vi "Stabilizing.vi"(4 "output cluster":T10, 5 "Max Humidity Wait Time":i32, 10 "output cluster 3":T2 {"Current Settings"."Pump" items=["Pump 0", "Pump 1", "Pump 2", "Pump 3", "Pump 4", "Pump 5"]; "Current Settings"."Chart X axis Timescale" min=20 max=180 step=1; "Current Settings"."RunTime Mode Settings"."Exp. Gas Tank" items=["0.07", "0.031", "0.877", "1.863", "3.881", "5.790", "7.688", "6.000"]; "Current Settings"."RunTime Mode Settings"."Insp. Gas Tank" items=["0.07", "0.031", "0.877", "1.863", "3.881", "5.790", "7.688", "6.000"]; "Current Settings"."RunTime Mode Settings"."I:E Ratio" max=30 scale=0.0..7.0; "Current Settings"."RunTime Mode Settings"."Resp Rate Brpm" min=0 max=30 format="%.2f"; "Current Settings"."TE#2 Configuration"."Serial Port"."XOFF Char" format="%.0x"; "Current Settings"."TE#2 Configuration"."Serial Port"."XON Char" format="%.0x"; "Current Settings"."TE#2 Configuration"."Serial Port"."flow control" items=["None"=0, "XON/XOFF"=1, "RTS/CTS"=2, "DTR/DSR"=4]; "Current Settings"."TE#2 Configuration"."Serial Port"."stop bits" items=["1.0"=10, "1.5"=15, "2.0"=20]; "Current Settings"."TE#2 Configuration"."Serial Port"."data bits" min=5 max=8 step=1; "Current Settings"."TE#2 Configuration"."Serial Port"."baud rate" items=["75"=75, "110"=110, "134"=134, "150"=150, "300"=300, "600"=600, "1200"=1200, "1800"=1800, "2400"=2400, "4800"=4800, "7200"=7200, "9600"=9600, "14400"=14400, "19200"=19200, "28800"=28800, "38400"=38400, "56000"=56000, "57600"=57600, "115200"=115200, "128000"=128000, "230400"=230400]; "Current Settings"."TE#2 Configuration"."Serial Port"."termination char" format="%.0x"; "Current Settings"."TE#1 Configuration"."Serial Port"."XOFF Char" format="%.0x"; "Current Settings"."TE#1 Configuration"."Serial Port"."XON Char" format="%.0x"; "Current Settings"."TE#1 Configuration"."Serial Port"."flow control" items=["None"=0, "XON/XOFF"=1, "RTS/CTS"=2, "DTR/DSR"=4]; "Current Settings"."TE#1 Configuration"."Serial Port"."stop bits" items=["1.0"=10, "1.5"=15, "2.0"=20]; "Current Settings"."TE#1 Configuration"."Serial Port"."data bits" min=5 max=8 step=1; "Current Settings"."TE#1 Configuration"."Serial Port"."baud rate" items=["75"=75, "110"=110, "134"=134, "150"=150, "300"=300, "600"=600, "1200"=1200, "1800"=1800, "2400"=2400, "4800"=4800, "7200"=7200, "9600"=9600, "14400"=14400, "19200"=19200, "28800"=28800, "38400"=38400, "56000"=56000, "57600"=57600, "115200"=115200, "128000"=128000, "230400"=230400]; "Current Settings"."TE#1 Configuration"."Serial Port"."termination char" format="%.0x"; "Current Settings"."Capnometer Configuration"."Device" items=["None", "TidalWave", "LoFlow / Canary", "Capnogard"]; "Current Settings"."Capnometer Configuration"."Serial Port"."XOFF Char" format="%.0x"; "Current Settings"."Capnometer Configuration"."Serial Port"."XON Char" format="%.0x"; "Current Settings"."Capnometer Configuration"."Serial Port"."flow control" items=["None"=0, "XON/XOFF"=1, "RTS/CTS"=2, "DTR/DSR"=4]; "Current Settings"."Capnometer Configuration"."Serial Port"."stop bits" items=["1.0"=10, "1.5"=15, "2.0"=20]; "Current Settings"."Capnometer Configuration"."Serial Port"."data bits" min=5 max=8 step=1; "Current Settings"."Capnometer Configuration"."Serial Port"."baud rate" items=["75"=75, "110"=110, "134"=134, "150"=150, "300"=300, "600"=600, "1200"=1200, "1800"=1800, "2400"=2400, "4800"=4800, "7200"=7200, "9600"=9600, "14400"=14400, "19200"=19200, "28800"=28800, "38400"=38400, "56000"=56000, "57600"=57600, "115200"=115200, "128000"=128000, "230400"=230400]; "Current Settings"."Capnometer Configuration"."Serial Port"."termination char" format="%.0x"; "Current Settings"."DAQx Settings"."Analog Output Settings (Volts)" format="%#.3g"; "Current Settings"."DAQx Settings"."Duty Cycle" min=10.0 max=90.0 format="%.1g"; "Current Settings"."DAQx Settings"."Frequency" min=20.0 max=200.0; "Current Settings"."DataLogging Settings"."Data File Duration (Minutes)" min=2 max=200 format="%#.2g"; "Current Settings"."Calibration Settings"."Tolerance #2" min=2 max=4096; "Current Settings"."Calibration Settings"."Cal. Average" min=2 max=4096; "Current Settings"."Test Settings"."Test Sensor ID" items=["(select)", "RB", "YC", "", "Other"]}, 11 "CalStatus":T1(ring)) -> (3 "NewCalStatus":T1(ring))   [LabVIEW 2016]
uses:
  Controls/Cal Refs.ctl
  Controls/DAQ Needed.ctl
  Controls/Processed Variables.ctl
  Controls/AirPump Controls.ctl
  Controls/IE Ratio knob.ctl
  Controls/UI Settings.ctl
  Controls/Aux CO2 Control.ctl
  Controls/Serial Visa Control.ctl
  Controls/Aux CO2 Selector.ctl
  Controls/Aux TE Control.ctl
  Controls/Queues And Others.ctl
  <vilib>/Analysis/baseanly.llb/Mean (DBL).vi
  <vilib>/Analysis/NI_AALBase.lvlib
panel:
  # "Note: Setting Brpm to zero will\ndisable Insp / Exp digital output."
  # "mmHg"
  # "pts"
  # "tolerance"
  # "AN5 (Temp 1)"
  # "AN6 (Temp 2)"
  # "AN7 (Temp 3)"
  # "AN8 (T FET)"
  # "AN0 (T POT)"
  # "Tref (Set Pt))"
  # "(Spare)"
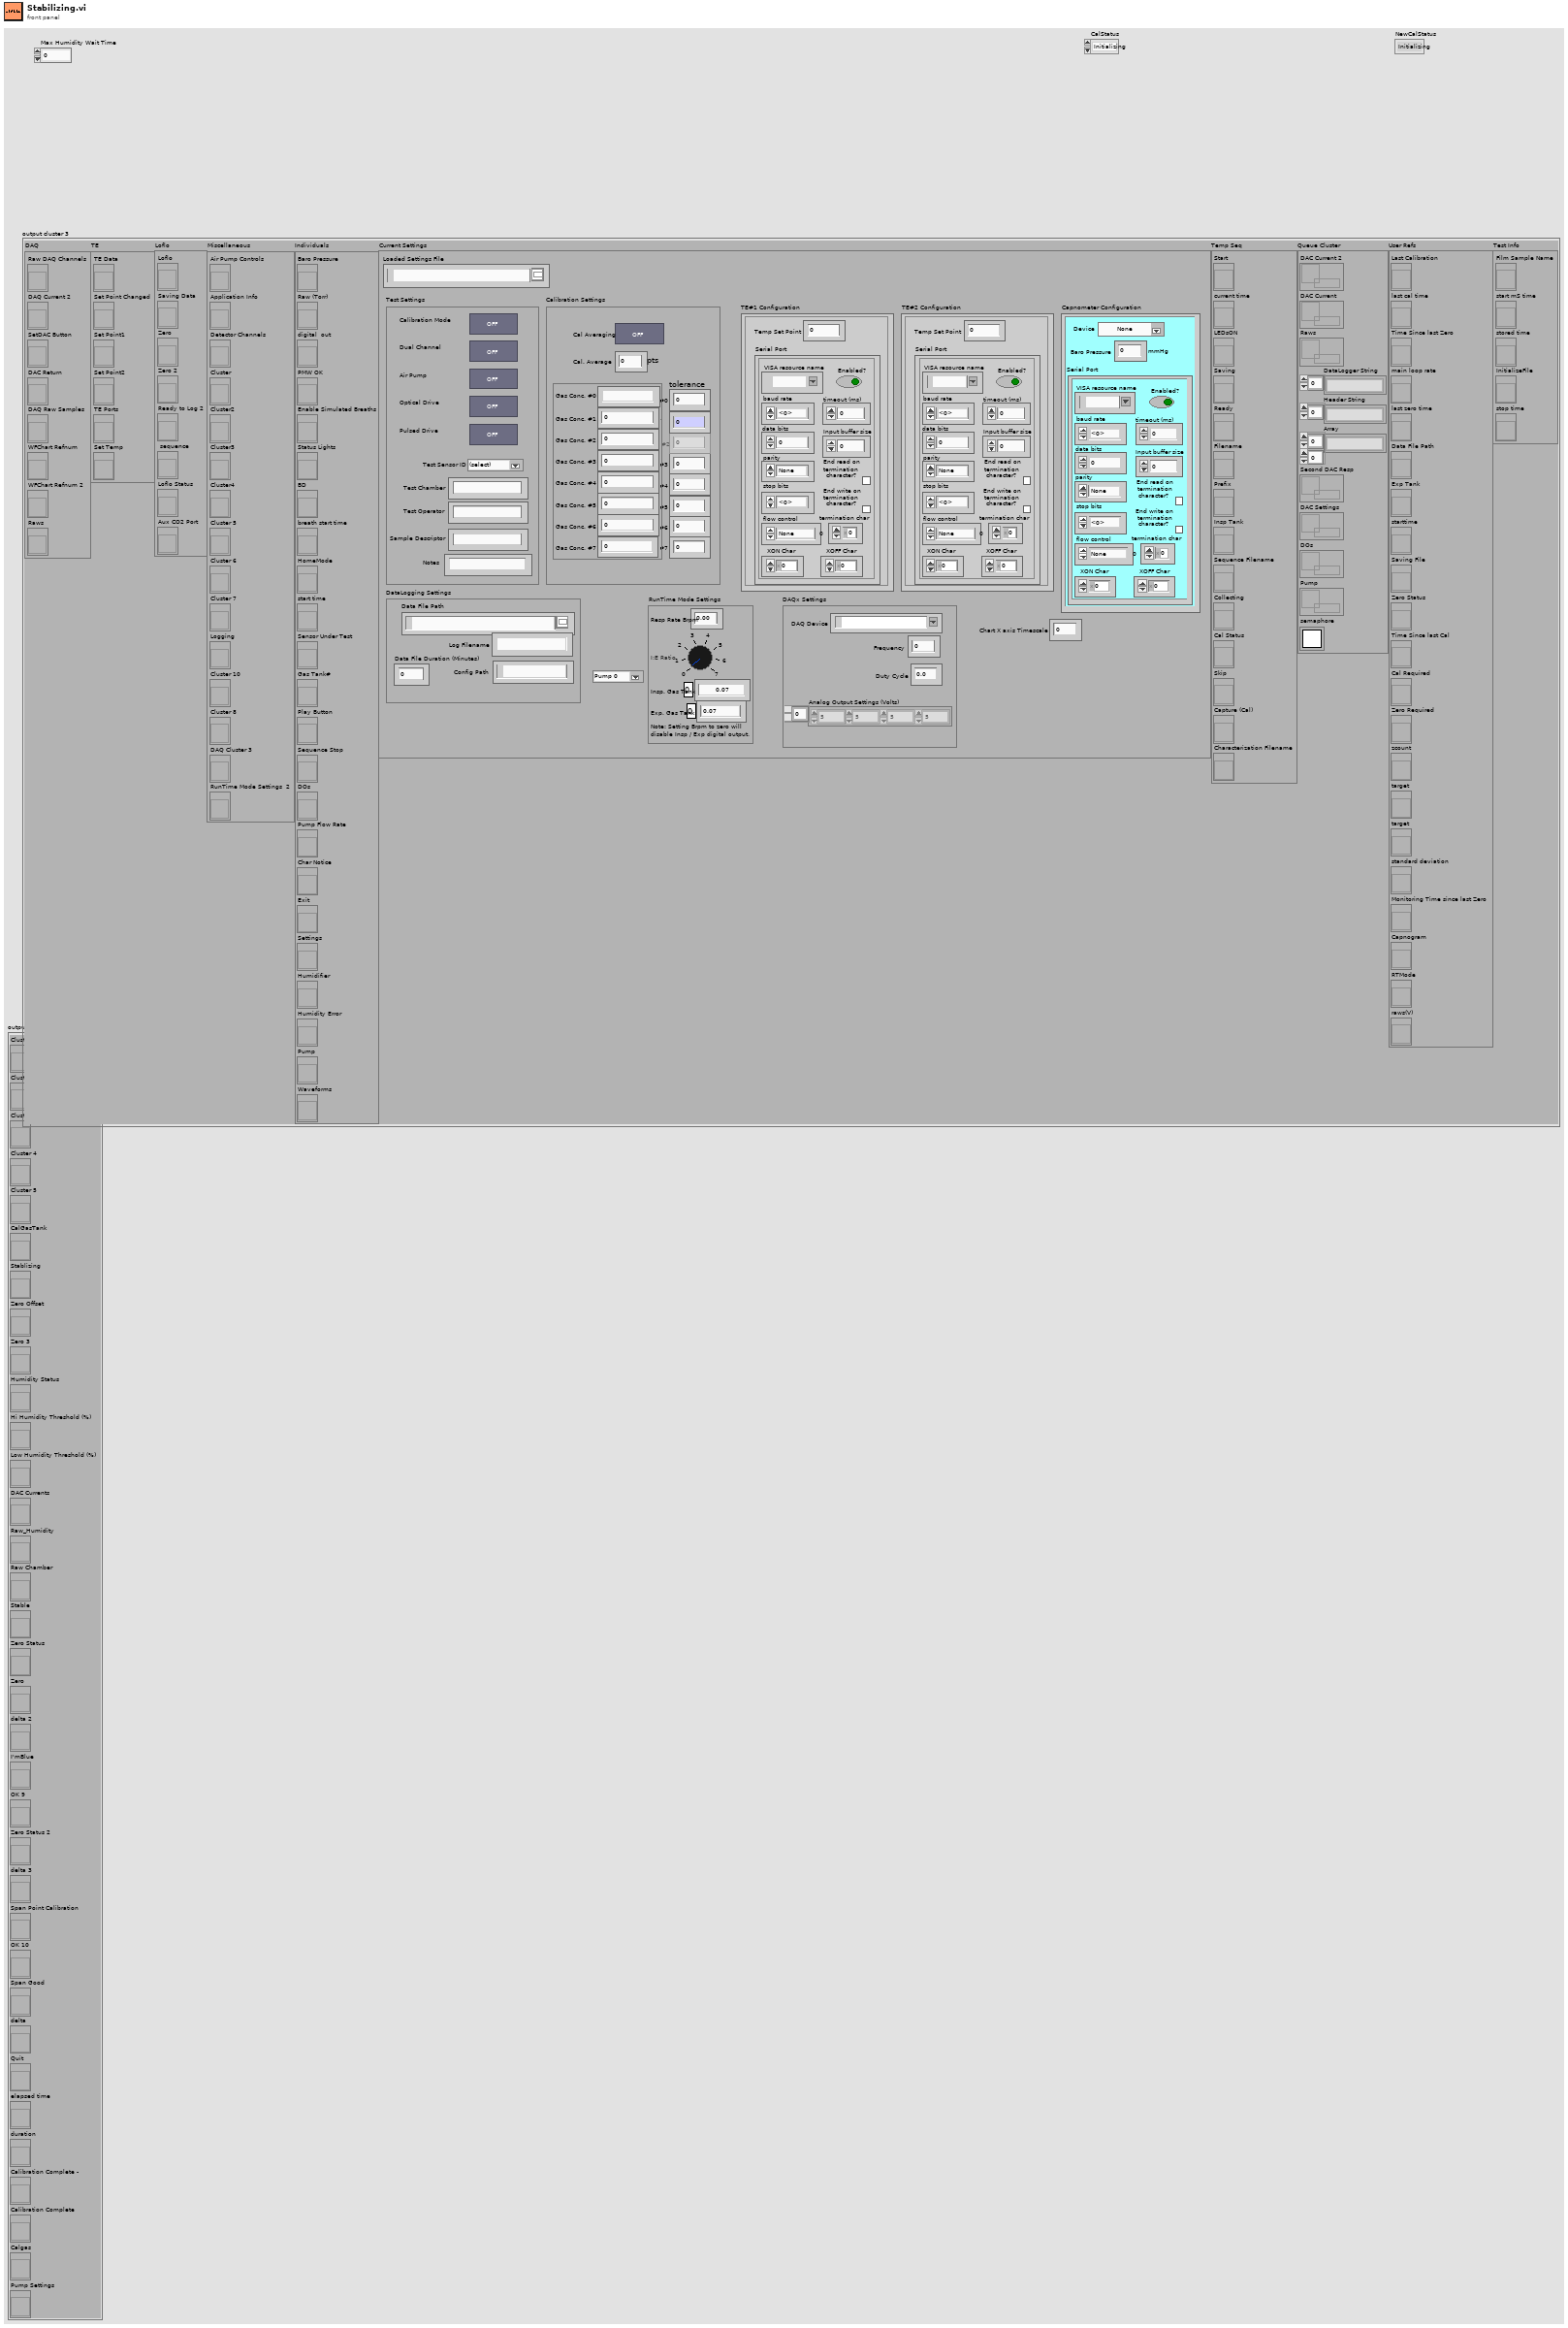
[diagram p1: front panel]
types:
  T1 = enum32{"Initializing", "Enter CO2 Value", "Enter Calibration Code", "Reading Calibration Data", "Stablizing", "Calculating Target Voltages", "Setting Zero Point", "Setting High Point", "Setting Span Point", "Calculating Gain & Offset", "Storing Calibration Coefficients", "Calibration Complete"}
  T2 = typedef "DAQ Needed.ctl" = cluster{"DAQ":cluster{"Raw DAQ Channels":refnum<vi>, "DAQ Current 2":refnum<vi>, "SetDAC Button":refnum<vi>, "DAC Return":refnum<vi>, "DAQ Raw Samples":refnum<vi>, "WFChart Refnum":refnum<vi>, "WFChart Refnum 2":refnum<vi>, "Raws":refnum<vi>}, "TE":cluster{"TE Data":refnum<vi>, "Set Point Changed":refnum<vi>, "Set Point1":refnum<vi>, "Set Point2":refnum<vi>, "TE Ports":refnum<vi>, "Set Temp":refnum<vi>}, "Loflo":cluster{"Loflo":refnum<vi>, "Saving Data":refnum<vi>, "Zero":refnum<vi>, "Zero 2":refnum<vi>, "Ready to Log 2":refnum<vi>, " sequence":refnum<vi>, "Loflo Status ":refnum<vi>, "Aux CO2 Port":refnum<vi>}, "Miscellaneous":cluster{"Air Pump Controls":refnum<vi>, "Application Info":refnum<vi>, "Detector Channels ":refnum<vi>, "Cluster":refnum<vi>, "Cluster2":refnum<vi>, "Cluster3":refnum<vi>, "Cluster4":refnum<vi>, "Cluster 5":refnum<vi>, "Cluster 6":refnum<vi>, "Cluster 7":refnum<vi>, "Logging":refnum<vi>, "Cluster 10":refnum<vi>, "Cluster 8":refnum<vi>, "DAQ Cluster 3":refnum<vi>, "RunTime Mode Settings  2":refnum<vi>}, "Individuals":cluster{"Baro Pressure":refnum<vi>, "Raw (Torr)":refnum<vi>, "digital  out":refnum<vi>, "PMW OK":refnum<vi>, "Enable Simulated Breaths":refnum<vi>, "Status Lights":refnum<vi>, "BD":refnum<vi>, "breath start time":refnum<vi>, "HomeMode":refnum<vi>, "start time":refnum<vi>, "Sensor Under Test":refnum<vi>, "Gas Tank#":refnum<vi>, "Play Button":refnum<vi>, "Sequence Stop":refnum<vi>, "DOs":refnum<vi>, "Pump Flow Rate":refnum<vi>, "Char Notice":refnum<vi>, "Exit":refnum<vi>, "Settings":refnum<vi>, "Humidifier":refnum<vi>, "Humidity Error":refnum<vi>, "Pump":refnum<vi>, "Waveforms":refnum<vi>}, "Current Settings":T3, "Temp Seq":cluster{"Start":refnum<vi>, "current time":refnum<vi>, "LEDsON":refnum<vi>, "Saving":refnum<vi>, "Ready":refnum<vi>, "Filename":refnum<vi>, "Prefix":refnum<vi>, "Insp Tank":refnum<vi>, "Sequence Filename":refnum<vi>, "Collecting":refnum<vi>, "Cal Status":refnum<vi>, "Skip":refnum<vi>, "Capture (Cal)":refnum<vi>, "Characterization Filename":refnum<vi>}, "Queue Cluster":T8, "User Refs":cluster{"Last Calibration":refnum<vi>, "last cal time":refnum<vi>, "Time Since last Zero":refnum<vi>, "main loop rate":refnum<vi>, "last zero time":refnum<vi>, "Data File Path":refnum<vi>, "Exp Tank":refnum<vi>, "starttime":refnum<vi>, "Saving File":refnum<vi>, "Zero Status":refnum<vi>, "Time Since last Cal":refnum<vi>, "Cal Required":refnum<vi>, "Zero Required":refnum<vi>, "zcount":refnum<vi>, "target":refnum<vi>, "target":refnum<vi>, "standard deviation":refnum<vi>, "Monitoring Time since last Zero":refnum<vi>, "Capnogram":refnum<vi>, "RTMode":refnum<vi>, "raws(V)":refnum<vi>}, "Test Info":cluster{"Film Sample Name":refnum<vi>, "start mS time":refnum<vi>, "stored time":refnum<vi>, "InitializeFile":refnum<vi>, "stop time":refnum<vi>}}
  T3 = typedef "UI Settings.ctl" = cluster{"Loaded Settings File":path, "Test Settings":cluster{"Dual Channel":bool, "Air Pump":bool, "Optical Drive":bool, "Pulsed Drive":bool, "Calibration Mode":bool, "Test Sensor ID":u16, "Test Chamber":string, "Test Operator":string, "Sample Descriptor":string, "Notes":string}, "Calibration Settings":cluster{"Cal. Average":u16, "Cal Averaging":bool, "Tolerance #0":sgl, "Tolerance #7":sgl, "Tolerance #6":sgl, "Tolerance #5":sgl, "Tolerance #4":sgl, "Tolerance #3":sgl, "Tolerance #2":sgl, "Tolerance #1":sgl, "Gas Tank Settings":cluster{"Gas Conc. #0":string, "Gas Conc. #1":sgl, "Gas Conc. #2":sgl, "Gas Conc. #3":sgl, "Gas Conc. #4":sgl, "Gas Conc. #5":sgl, "Gas Conc. #6":sgl, "Gas Conc. #7":sgl}}, "DataLogging Settings":cluster{"Data File Path":path, "Data File Duration (Minutes)":sgl, "Log Filename":string, "Config Path":path}, "DAQx Settings":cluster{"DAQ Device":tag, "Frequency":dbl, "Duty Cycle":dbl, "Analog Output Settings (Volts)":sgl[]}, "Capnometer Configuration":T4, "TE#1 Configuration":T7, "TE#2 Configuration":T7, "RunTime Mode Settings ":cluster{"Resp Rate Brpm ":sgl, "I:E Ratio":u8, "Insp. Gas Tank":u16, "Exp. Gas Tank":u16}, "Chart X axis Timescale":u16, "Pump":u16}
  T4 = typedef "Aux CO2 Control.ctl" = cluster{"Serial Port":T5, "Baro Pressure":u32, "Device":T6}
  T5 = typedef "Serial Visa Control.ctl" = cluster{"termination char":u8, "End read on termination character?":bool, "Enabled?":bool, "VISA resource name":refnum<visa-resource-name>, "baud rate":u32, "data bits":u16, "parity":enum16{"None", "Odd", "Even", "Mark", "Space"}, "stop bits":u16, "flow control":u16, "timeout (ms)":u32, "Input buffer size":u32, "End write on termination character?":bool, "XON Char":u8, "XOFF Char":u8}
  T6 = typedef "Aux CO2 Selector.ctl" = u16
  T7 = typedef "Aux TE Control.ctl" = cluster{"Temp Set Point":sgl, "Serial Port":T5}
  T8 = typedef "Queues And Others.ctl" = cluster{"DAC Current 2":refnum<queue>, "DAC Current":refnum<queue>, "Raws":refnum<queue>, "DataLogger String":string[], "Header String":string[], "Array":string[][], "Second DAC Resp":refnum<queue>, "DAC Settings":refnum<queue>, "DOs":refnum<queue>, "Pump":refnum<queue>, "semaphore":T9}
  T9 = typedef "Semaphore RefNum" = refnum<k1>
  T10 = typedef "Cal Refs.ctl" = cluster{"Cluster":refnum<vi>, "Cluster 2":refnum<vi>, "Cluster 3":refnum<vi>, "Cluster 4":refnum<vi>, "Cluster 5":refnum<vi>, "CalGasTank":refnum<vi>, "Stablizing":refnum<vi>, "Zero Offset":refnum<vi>, "Zero 3":refnum<vi>, "Humidity Status":refnum<vi>, "Hi Humidity Threshold (%)":refnum<vi>, "Low Humidity Threshold (%)":refnum<vi>, "DAC Currents":refnum<vi>, "Raw_Humidity":refnum<vi>, "Raw Chamber":refnum<vi>, "Stable":refnum<vi>, "Zero Status":refnum<vi>, "Zero":refnum<vi>, "delta 2":refnum<vi>, "I'mBlue":refnum<vi>, "OK 9":refnum<vi>, "Zero Status 2":refnum<vi>, "delta 3":refnum<vi>, "Span Point Calibration":refnum<vi>, "OK 10":refnum<vi>, "Span Good":refnum<vi>, "delta":refnum<vi>, "Quit":refnum<vi>, "elapsed time":refnum<vi>, "duration":refnum<vi>, "Calibration Complete -":refnum<vi>, "Calibration Complete":refnum<vi>, "Calgas":refnum<vi>, "Pump Settings":refnum<vi>}
  T11 = enum16{"Waiting For Film to Stabilize", "Film Stable", "Exiting", "Initializing"}
  T12 = enum16{"Waiting For Film to Stabilize", "Film Stable - Press OK to Continue", "Exiting"}
  T13 = enum16{"Waiting For Film to Stabilize", "Film Stable - Press OK to Continue", "Exiting", "Initializing"}
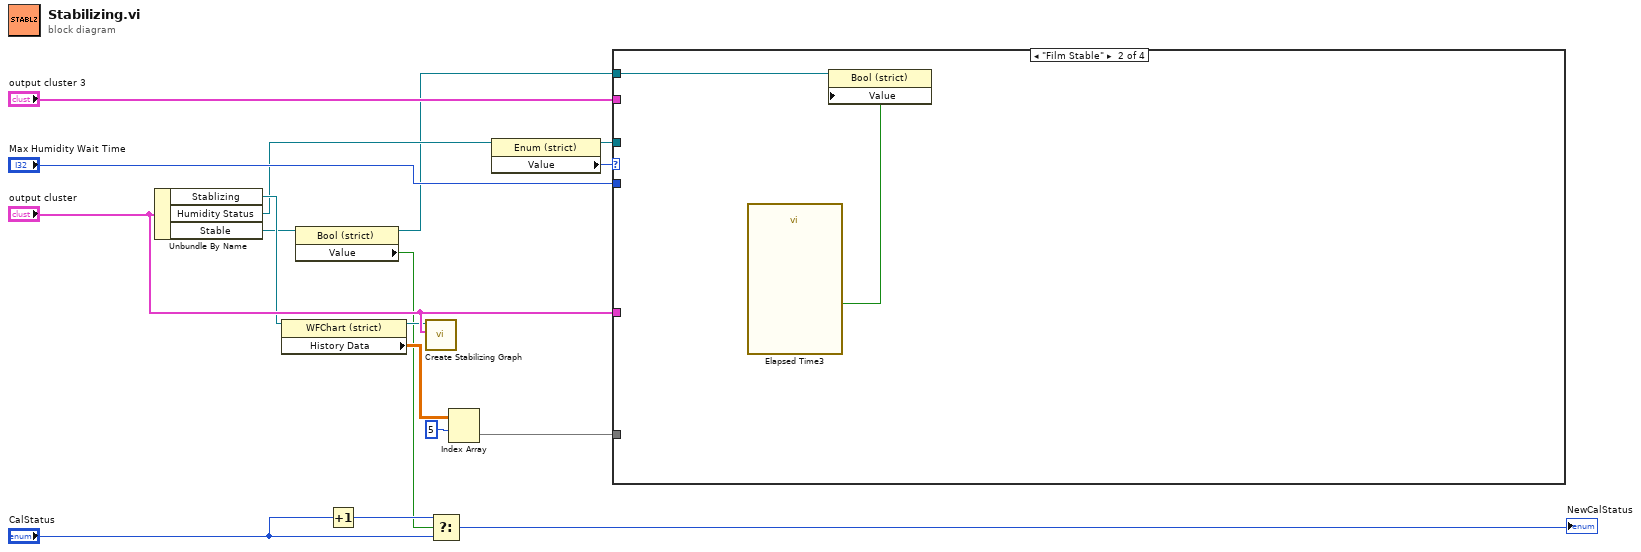
[diagram p0: block diagram]
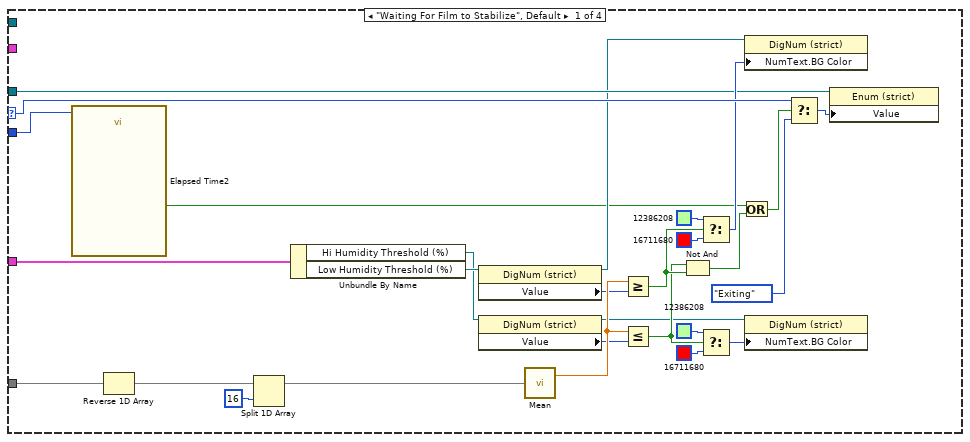
[diagram p2: hidden frame]
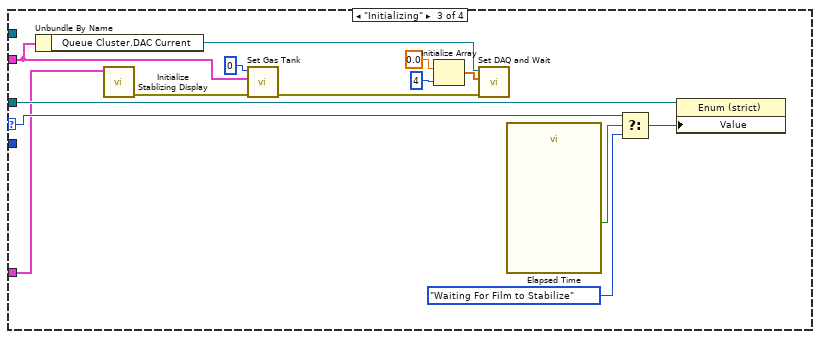
[diagram p3: hidden frame]
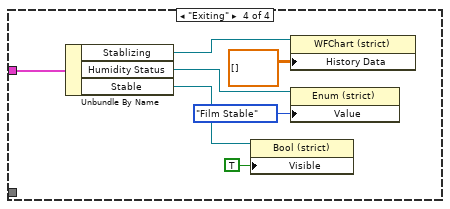
[diagram p4: hidden frame]
diagram:
  n1 = Unbundle By Name("output cluster") -> ("Stablizing"=w11:refnum<vi>, "Humidity Status"=w7:refnum<vi>, "Stable"=w6:refnum<vi>)
  n2 = property on="Property Node" class="WFChart (strict)"(reference=w11) -> (reference out=w10:refnum<vi>, "History Data"=w13:dbl[][])  [unwired: 1 in, 1 out]
  n3 = property on="Property Node" class="Bool (strict)"(reference=w6) -> (reference out=w5:refnum<vi>, "Value"=w9:bool)  [unwired: 1 in, 1 out]
  n4 = Increment(x="CalStatus") -> (x+1=w12:T1)
  n5 = call "Create Stabilizing Graph.vi"("output cluster"="output cluster", "WaveformChart in"=w10) -> ()  [unwired: 9 in, 1 out]
  n6 = Select(t=w12, s=w9, f="CalStatus") -> (s? t:f=→"NewCalStatus":T1)
  n7 = Index Array(array=w13, index (row)=5) -> (element=w4:dbl[])  [unwired: 1 in]
  n8 = property class="Enum (strict)"(reference=w7) -> (reference out=w3:refnum<vi>, "Value"=w8:T11)  [unwired: 1 in, 1 out]
  n9 = case shown="\"Film Stable\"" w8 {
    selector: w8 -> [w45 _ w60 _]
    tunnel: "Max Humidity Wait Time" -> [w21 _ _ _]
    tunnel: w5 -> [_ w47 _ _]
    tunnel: w3 -> [w35 _ w59 _]
    tunnel: w4 -> [w30 _ _ _]
    tunnel: "output cluster" -> [w26 _ w49 w65]
    tunnel: "output cluster 3" -> [_ _ w50 _]
    frame "Waiting For Film to Stabilize", Default {
      n10 = call "Elapsed Time2"("Time Target (s)"=w21) -> ("Time has Elapsed"=w20:bool)  [unwired: 11 in, 7 out]
      n11 = Reverse 1D Array(array=w30) -> (reversed array=w29:dbl[])
      n12 = Split 1D Array(array=w29, index=16) -> (first subarray=w31:dbl[])  [unwired: 1 out]
      n13 = Unbundle By Name(w26) -> ("Hi Humidity Threshold (%)"=w24:refnum<vi>, "Low Humidity Threshold (%)"=w25:refnum<vi>)
      n14 = property class="DigNum (strict)"(reference=w25) -> (reference out=w28:refnum<vi>, "Value"=w27:u16)  [unwired: 1 in, 1 out]
      n15 = property class="DigNum (strict)"(reference=w24) -> (reference out=w23:refnum<vi>, "Value"=w22:u16)  [unwired: 1 in, 1 out]
      n16 = call-poly <vilib>:"Mean.vi"("X"=w31) -> ("mean"=w33:dbl)  [unwired: 1 out]
      n17 = Greater Or Equal?(x=w33, y=w27) -> (x >= y?=w42:bool)
      n18 = Less Or Equal?(x=w33, y=w22) -> (x <= y?=w40:bool)
      n19 = Not And(1:w42, 2:w40) -> (0:w19:bool)
      n20 = Select(t=u32 12386208, s=w42, f=u32 16711680) -> (s? t:f=w43:u32)
      n21 = Select(t=u32 12386208, s=w40, f=u32 16711680) -> (s? t:f=w41:u32)
      n22 = Or(x=w20, y=w19) -> (x .or. y?=w18:bool)
      n23 = property on="Property Node" class="DigNum (strict)"(reference=w28, "NumText.BG Color"=w43) -> ()  [unwired: 1 in, 2 out]
      n24 = property on="Property Node" class="DigNum (strict)"(reference=w23, "NumText.BG Color"=w41) -> ()  [unwired: 1 in, 2 out]
      n25 = Select(t=w45, s=w18, f=T12."Exiting" ("Humidity Status")) -> (s? t:f=w34:u16)
      n26 = property class="Enum (strict)"(reference=w35, "Value"=w34) -> ()  [unwired: 1 in, 2 out]
    }
    frame "Film Stable" {
      n27 = call "Elapsed Time3"() -> ("Time has Elapsed"=w46:bool)  [unwired: 12 in, 7 out]
      n28 = property on="Property Node" class="Bool (strict)"(reference=w47, "Value"=w46) -> ()  [unwired: 1 in, 2 out]
    }
    frame "Initializing" {
      n29 = Unbundle By Name(w50) -> ("Queue Cluster.DAC Current"=w57:refnum<queue>)
      n30 = call "Initialize Stablizing Display.vi"("output cluster"=w49) -> ("error out"=w51:errorcluster)  [unwired: 9 in, 1 out]
      n31 = call "Set Gas Tank.vi"("error in (no error)"=w51, "input cluster"=w50, "Gas Tank"=u8 0 ("CalGasTank")) -> ("error out"=w52:errorcluster)  [unwired: 7 in, 1 out]
      n32 = Initialize Array(0.0, 4 ("dimension size")) -> (w53:dbl[])
      n33 = call "Set DAQ and Wait.vi"("error in (no error)"=w52, "Array"=w53, "Queue in"=w57) -> ()  [unwired: 9 in]
      n34 = call "Elapsed Time"() -> ("Time has Elapsed"=w48:bool)  [unwired: 12 in, 7 out]
      n35 = Select(t=w60, s=w48, f=T13."Waiting For Film to Stabilize" ("Humidity Status")) -> (s? t:f=w58:u16)
      n36 = property class="Enum (strict)"(reference=w59, "Value"=w58) -> ()  [unwired: 1 in, 2 out]
    }
    frame "Exiting" {
      n37 = Unbundle By Name(w65) -> ("Stablizing"=w64:refnum<vi>, "Humidity Status"=w63:refnum<vi>, "Stable"=w62:refnum<vi>)
      n38 = property on="Property Node" class="Bool (strict)"(reference=w62, "Visible"=TRUE) -> ()  [unwired: 1 in, 2 out]
      n39 = property on="Property Node" class="WFChart (strict)"(reference=w64, "History Data"=dbl[][] []) -> ()  [unwired: 1 in, 2 out]
      n40 = property class="Enum (strict)"(reference=w63, "Value"=T11."Film Stable" ("Humidity Status")) -> ()  [unwired: 1 in, 2 out]
    }
  }
